vi "distribute shared data.vi"(8 "error in (no error)":errorcluster, 11 "Item Ref in":T1 format="%.0x") -> (0 "error out":errorcluster, 3 "Item Ref out":T1 format="%.0x")   [LabVIEW 2017, in "DSF System Explorer.lvlib"]
uses:
  DSF System Explorer.lvlib
  <vilib>/NI Veristand/Custom Device API/Custom Device Item Ref.ctl
  <vilib>/NI Veristand/Custom Device API/Custom Device API.lvlib
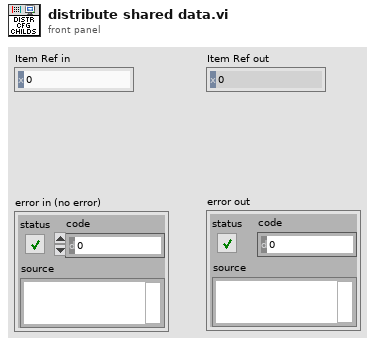
[diagram p1: front panel]
types:
  T1 = typedef "Custom Device API.lvlib/Custom Device Item Ref.ctl" = u64
  T2 = typedef "DSF System Explorer.lvlib/shared data ref.ctl" = refnum<data-value>
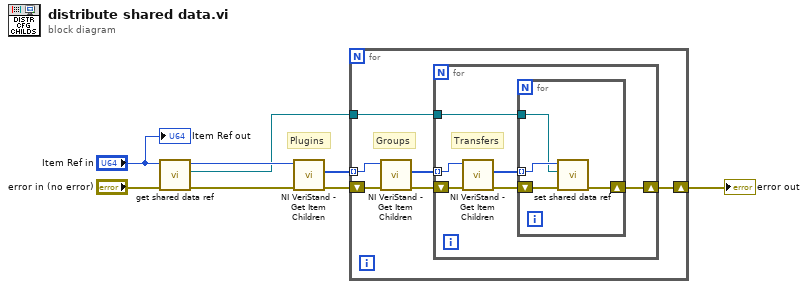
[diagram p0: block diagram]
diagram:
  # "Plugins"
  n1 = call "get shared data ref.vi"("error in (no error)"="error in (no error)", "Item Ref in"="Item Ref in") -> ("error out"=w7:errorcluster, "shared data ref"=w1:T2, "Item Ref out"=w3:T1)  [unwired: 7 in]
  n2 = call <vilib>:"NI VeriStand - Get Item Children.vi"("error in (no error)"=w7, "Item Ref in"=w3) -> ("error out"=w6:errorcluster, "Child Refs"=w5:T1[])  [unwired: 6 in, 2 out]
  n3 = for {
    shift-right: [w10] -> w4
    shift-left: w6 -> [w14]
    tunnel: w5 -> [w11] mode=indexing
    tunnel: w1 -> [w9]
    # "Groups"
    n4 = call <vilib>:"NI VeriStand - Get Item Children.vi"("error in (no error)"=w14, "Item Ref in"=w11) -> ("error out"=w12:errorcluster, "Child Refs"=w13:T1[])  [unwired: 6 in, 2 out]
    n5 = for {
      tunnel: w13 -> [w20] mode=indexing
      shift-right: [w16] -> w10
      shift-left: w12 -> [w19]
      tunnel: w9 -> [w15]
      # "Transfers"
      n6 = call <vilib>:"NI VeriStand - Get Item Children.vi"("error in (no error)"=w19, "Item Ref in"=w20) -> ("error out"=w18:errorcluster, "Child Refs"=w17:T1[])  [unwired: 6 in, 2 out]
      n7 = for {
        shift-right: [w22] -> w16
        shift-left: w18 -> [w24]
        tunnel: w17 -> [w23] mode=indexing
        tunnel: w15 -> [w21]
        n8 = call "set shared data ref.vi"("error in (no error)"=w24, "shared data ref"=w21, "Node Ptr"=w23) -> ("error out"=w22:errorcluster)  [unwired: 7 in, 1 out]
      }
    }
  }
  "error out" <- w4
  "Item Ref out" <- "Item Ref in"
